vi "Set Serial Number (z).vi"(8 "Error In":errorcluster, 10 "Serial Number":u16, 11 "VISA resource name in":refnum<visa-resource-name>) -> (0 "Error out":errorcluster, 1 "ACK":bool, 3 "VISA resource name out":refnum<visa-resource-name>)   [LabVIEW 2015]
uses:
  Ctls/Cmd str.ctl
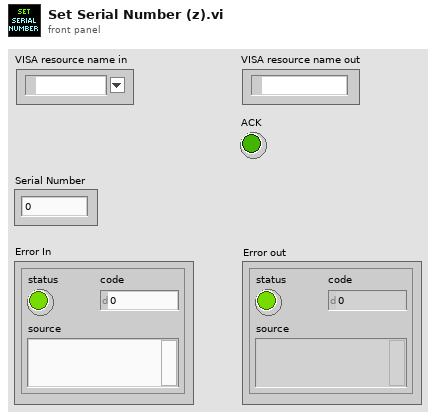
[diagram p1: front panel]
types:
  T1 = typedef "Cmd str.ctl" = string
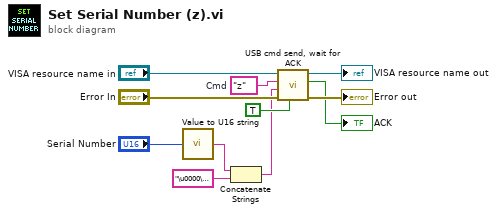
[diagram p0: block diagram]
diagram:
  w4 = T1 "z"  # Cmd
  n1 = call "Value to U16 string.vi"("Value"="Serial Number") -> ("U16 str (Little Endian)"=w3:string)
  n2 = Concatenate Strings(w3, "\u0000\u0000" ("string")) -> (w2:string)
  n3 = call "USB cmd send, wait for ACK.vi"("Wait for ACK?"=TRUE, "Error In"="Error In", "4 byte config str"=w2, "Cmd"=w4, "VISA resource name in"="VISA resource name in") -> ("Error out"=→"Error out":errorcluster, "ACK ok"=→"ACK":bool, "VISA resource name out"=→"VISA resource name out":refnum<visa-resource-name>)  [unwired: 1 in, 1 out]
